vi "BRig_RT__Case_Exp__UploadClosedLoop__v3.vi"() -> (2 "all rows":i64[][](array[numeric]), 3 "output_haveCmd":bool)   [LabVIEW 2014]
uses:
  <vilib>/Utility/file.llb/Read From Spreadsheet File (I64).vi
panel:
  out "received":bool
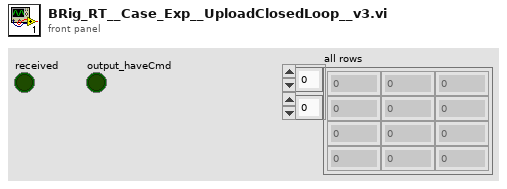
[diagram p1: front panel]
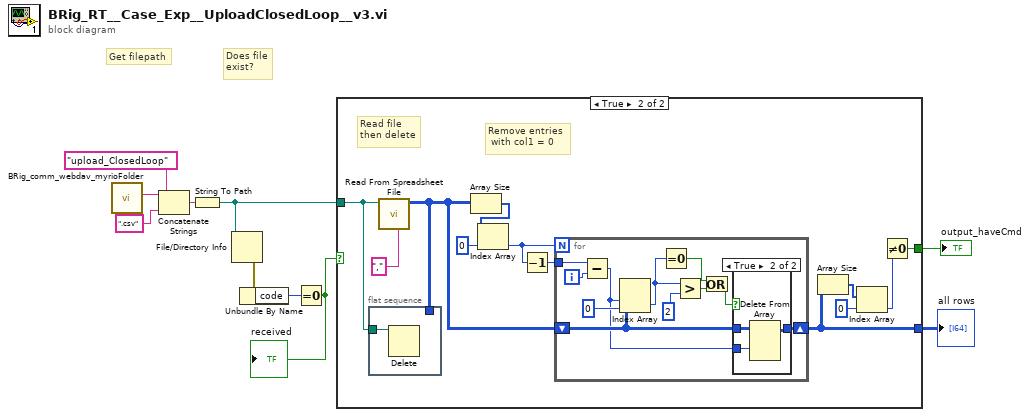
[diagram p0: block diagram]
diagram:
  # "Does file\nexist?"
  # "Get filepath"
  n1 = call "BRig_comm_webdav_myrioFolder.vi"() -> ("output_myrioFolder"=w3:string)  [unwired: 11 in]
  n2 = Concatenate Strings(w3, "upload_ClosedLoop" ("string"), ".csv" ("string")) -> (w10:string)
  n3 = String To Path(string=w10) -> (path=w4:path)
  n4 = File/Directory Info(path=w4) -> (error out=w7:errorcluster)  [unwired: 1 in, 6 out]
  n5 = Unbundle By Name(w7) -> ("code"=w6:i32)
  n6 = Equal To 0?(x=w6) -> (x = 0?=w5:bool)
  "received" <- w5
  n7 = case shown="True" w5 {
    tunnel: w4 -> [_ w22]
    tunnel: [_ w12] -> w2
    tunnel: [_ w11] -> w1
    frame False {
    }
    frame True {
      # "Remove entries\n with col1 = 0"
      # "Read file\nthen delete"
      n8 = flat-sequence {
        tunnel: w22 -> [w38]
        tunnel: w16 -> [_]
        frame #0 {
          n9 = Delete(path (use dialog)=w38) -> ()  [unwired: 4 in, 3 out]
        }
      }
      n10 = call-poly <vilib>:"Read From Spreadsheet File.vi"("delimiter (\\t)"="," ("delimiter (\\t)"), "file path (dialog if empty)"=w22) -> ("all rows"=w16:i64[][])  [unwired: 5 in, 4 out]
      n11 = Array Size(array=w16) -> (size(s)=w20:i32[])
      n12 = Index Array(array=w20, index=0) -> (element=w18:i32)
      n13 = Decrement(x=w18) -> (x-1=w17:i32)
      n14 = for {
        N: w18 -> [_]
        shift-right: [w29] -> w12
        shift-left: w16 -> [w30]
        tunnel: w17 -> [w33]
        i -> [w32]
        n15 = Subtract(x=w33, y=w32) -> (x-y=w28:i32)
        n16 = Index Array(array=w30, index (row)=w28, index (col)=0 ("disabled index (col)")) -> (element=w27:i64)
        n17 = Equal To 0?(x=w27) -> (x = 0?=w24:bool)
        n18 = Greater?(x=w27, y=i64 2) -> (0:w25:bool)
        n19 = Or(x=w24, y=w25) -> (x .or. y?=w23:bool)
        n20 = case shown="True" w23 {
          tunnel: w30 -> [w34 w37]
          tunnel: [w34 w36] -> w29
          tunnel: w28 -> [_ w35]
          frame False {
          }
          frame True {
            n21 = Delete From Array(array=w37, index (row)=w35) -> (array with subset deleted=w36:i64[][])  [unwired: 2 in, 1 out]
          }
        }
      }
      n22 = Array Size(array=w12) -> (size(s)=w14:i32[])
      n23 = Index Array(array=w14, index=0) -> (element=w13:i32)
      n24 = Not Equal To 0?(x=w13) -> (x != 0?=w11:bool)
    }
  }
  "output_haveCmd" <- w1
  "all rows" <- w2
